vi "Configure DC Voltage.vi"(0 "VISA resource name":refnum<visa-resource-name>, 1 "NPLC":u16(ring)=1 items=["0.00005", "1", "12", "15"], 2 "DB Reference":dbl=1.0 min=1e-07 max=1000.0, 5 "Auto Range? (T: Auto)":bool=TRUE, 7 "Manual Range":dbl=1000.0, 9 "Aperture Seconds":dbl, 11 "error in (no error)":errorcluster, 12 "Input Impedance (10 M Ohm)":u16(ring) items=["10 M Ohm", "Auto"], 13 "Unit":u16(ring) items=["Volt", "DB"]) -> (4 "VISA resource name out":refnum<visa-resource-name>, 15 "error out":errorcluster)   [LabVIEW 2017, in "Keithley DMM7510.lvlib"]
doc: "This VI configures the DC Voltage measurement and the related parameters."
uses:
  Keithley DMM7510.lvlib
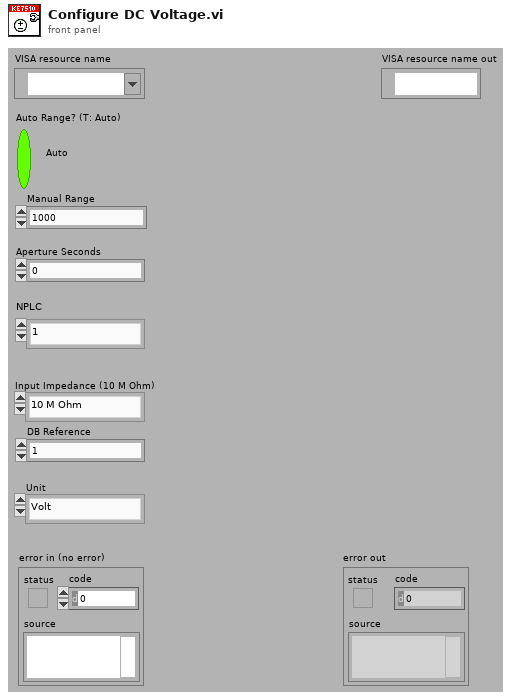
[diagram p1: front panel]
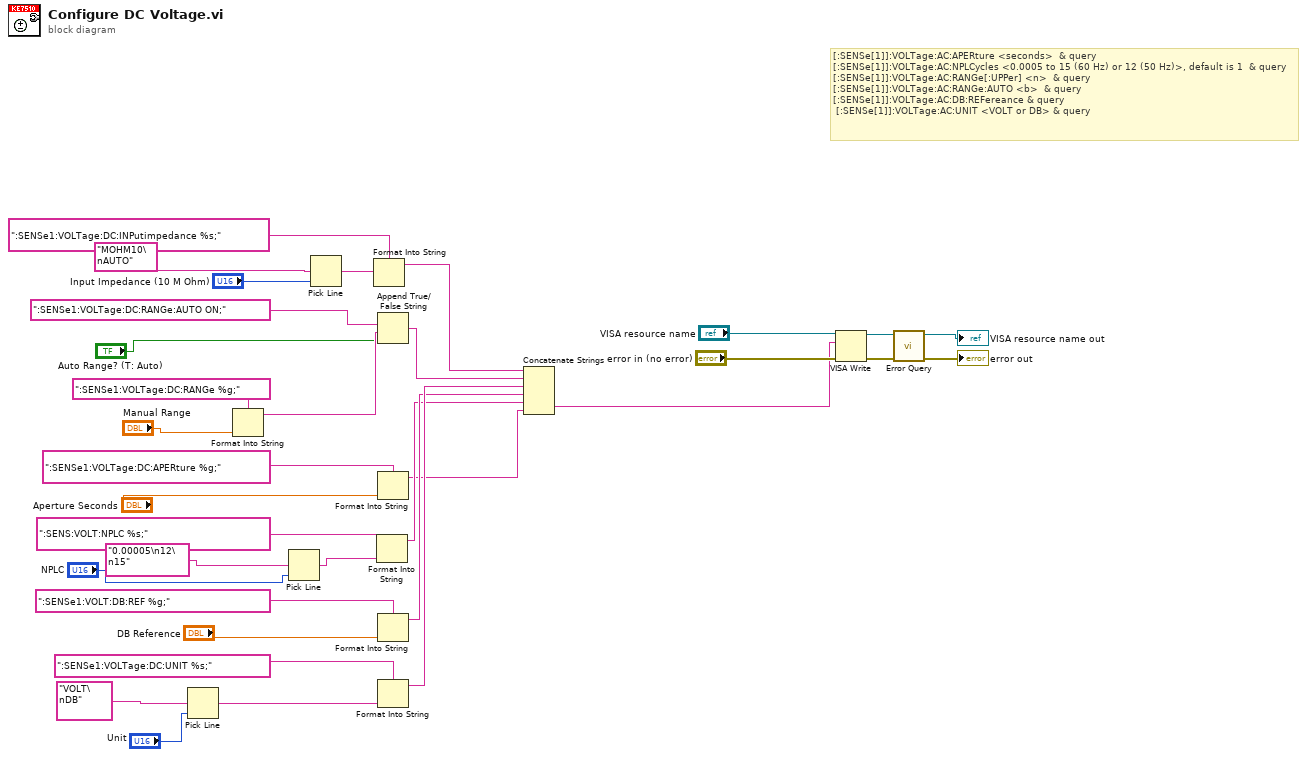
[diagram p0: block diagram]
diagram:
  # "[:SENSe[1]]:VOLTage:AC:APERture <seconds>  & query\n[:SENSe[1]]:VOLTage:AC:NPLCycles <0.0005 to 15 (60 Hz) or 12 (50 Hz)>, default is 1  & query\n[:SENSe[1]]:VOLTage:AC:RANGe[:UPPer] <n>  & query\n[:SENSe[1]]:VOLTage:AC:RANGe:AUTO <b>  & query\n[:SENSe[1]]:VOLTage:AC:DB:REFereance & query\n [:SENSe[1]]:VOLTage:AC:UNIT <VOLT or DB> & query"
  n1 = Pick Line(multi-line string="VOLT\nDB", line index="Unit") -> (output string=w19:string)  [unwired: 1 in]
  n2 = Format Into String(format string=":SENSe1:VOLTage:DC:RANGe %g;", "Manual Range") -> (resulting string=w29:string)  [unwired: 2 in, 1 out]
  n3 = Pick Line(multi-line string="0.00005\n12\n15", line index="NPLC") -> (output string=w9:string)  [unwired: 1 in]
  n4 = Pick Line(multi-line string="MOHM10\nAUTO", line index="Input Impedance (10 M Ohm)") -> (output string=w12:string)  [unwired: 1 in]
  n5 = Format Into String(format string=":SENSe1:VOLTage:DC:INPutimpedance %s;", w12) -> (resulting string=w26:string)  [unwired: 2 in, 1 out]
  n6 = Format Into String(format string=":SENS:VOLT:NPLC %s;", w9) -> (resulting string=w2:string)  [unwired: 2 in, 1 out]
  n7 = Append True/False String(1:"Auto Range? (T: Auto)", 2:w29, 3:":SENSe1:VOLTage:DC:RANGe:AUTO ON;") -> (0:w25:string)  [unwired: 1 in]
  n8 = Format Into String(format string=":SENSe1:VOLTage:DC:APERture %g;", "Aperture Seconds") -> (resulting string=w1:string)  [unwired: 2 in, 1 out]
  n9 = Format Into String(format string=":SENSe1:VOLT:DB:REF %g;", "DB Reference") -> (resulting string=w3:string)  [unwired: 2 in, 1 out]
  n10 = Format Into String(format string=":SENSe1:VOLTage:DC:UNIT %s;", w19) -> (resulting string=w4:string)  [unwired: 2 in, 1 out]
  n11 = Concatenate Strings(w26, w25, w4, w3, w2, w1) -> (w24:string)
  n12 = VISA Write(VISA resource name="VISA resource name", write buffer=w24, error in (no error)="error in (no error)") -> (VISA resource name out=w17:refnum<visa-resource-name>, error out=w16:errorcluster)  [unwired: 1 out]
  n13 = call "Error Query.vi"("error in (no error)"=w16, "VISA resource name"=w17) -> ("error out"=→"error out":errorcluster, "VISA resource name out"=→"VISA resource name out":refnum<visa-resource-name>)  [unwired: 6 in, 2 out]
